vi "Mcp2210 Set Permanent Lock.vi"(8 "error in (no error)":errorcluster, 11 "handle":i32) -> (0 "error out":errorcluster, 3 "handle out":i32)   [LabVIEW 2015, in "mcp2210.lvlib"]
doc: "Permanently locks the device NVRAM settings.\n!!!!!!!!!!!!!!!!!!!!!!!!!!!!!!!! WARNING !!!!!!!!!!!!!!!!!!!!!!!!!!!!!!!!!!!\nUSE THIS FUNCTION WITH GREAT CAUTION. THERE IS NO WAY TO REMOVE THE PERMANENT LOCK\nTHE CHIP POWER-UP DEFAULT SETTINGS CANNOT BE CHANGED AFTER THIS FUNCTION CALL\n!!!!!!!!!!!!!!!!!!!!!!!!!!!!!!!!!!!!!!!!!!!!!!!!!!!!!!!!!!!!!!!!!!!!!!!!!!!!!!!!!!\nThe function returns 0 (M_E_SUCCESS) if the lock configuration is accepted\nor negative error code in case of device communication failure or if the access control configuration\nchange is not accepted by the device.\nError codes in case of rejected configuration change:\n- M_E_ERR_NVRAM_LOCKED - NVRAM is already permanently locked\n- M_E_ERR_BLOCKED_ACCESS - NVRAM is password protected. NVRAM change protection must be\ndeactivated first, using M_Mcp2210_EnterPassword() or\nM_Mcp2210_SetAccessControl()\nParameters:\nInputs:\n- IntPtr handle - The USB device handle. Cannot be NULL.\nOutputs:\n- none\nReturns:\n- 0 for success: M_E_SUCCESS\n- negative error code: M_E_ERR_NULL, M_E_ERR_INVALID_HANDLE_VALUE, M_E_ERR_INVALID_PARAMETER\nM_E_ERR_HID_TIMEOUT, M_E_ERR_HID_RW_FILEIO, M_E_ERR_UNKOWN_ERROR\nM_E_ERR_NVRAM_LOCKED, M_E_ERR_BLOCKED_ACCESS\nM_E_ERR_CMD_ECHO, M_E_ERR_CMD_FAILED\n\nMCP2210_DLL_UM_API int __stdcall Mcp2210_SetPermanentLock(void *handle);"
uses:
  <userlib>/mcp2210/mcp2210.lvlib
  <userlib>/mcp2210/mcp2210_dll_um_x86.dll
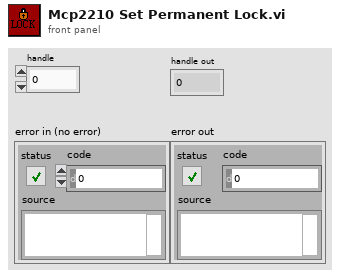
[diagram p1: front panel]
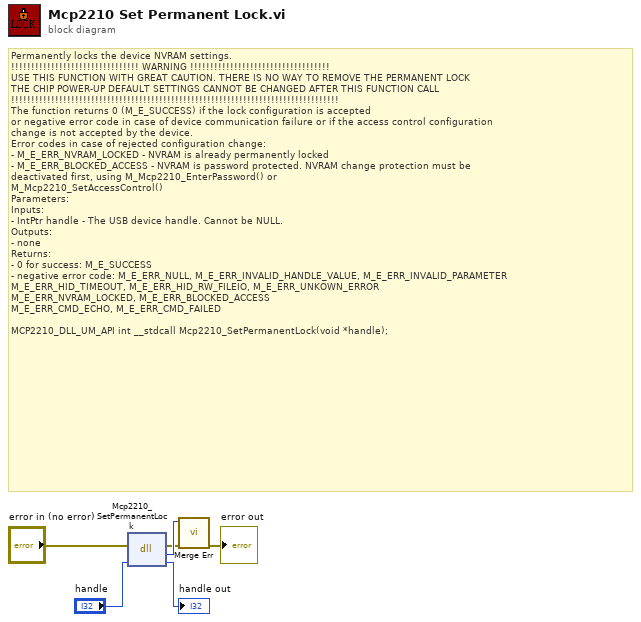
[diagram p0: block diagram]
diagram:
  # "Permanently locks the device NVRAM settings.\n!!!!!!!!!!!!!!!!!!!!!!!!!!!!!!!! WARNING !!!!!!!!!!!!!!!!!!!!!!!!!!!!!!!!!!!\nUSE THIS FUNCTION WITH GREAT CAUTION. THERE IS NO WAY TO REMOVE THE PERMANENT LOCK\nTHE CHIP POWER-UP DEFAULT SETTINGS CANNOT BE CHANGED AFTER THIS FUNCTION CALL\n!!!!!!!!!!!!!!!!!!!!!!!!!!!!!!!!!!!!!!!!!!!!!!!!!!!!!!!!!!!!!!!!!!!!!!!!!!!!!!!!!!\nThe function returns 0 (M_E_SUCCESS) if the lock configuration is accepted\nor negative error code in case of device communication failure or if the access control configuration\nchange is not accepted by the device.\nError codes in case of rejected configuration change:\n- M_E_ERR_NVRAM_LOCKED - NVRAM is already permanently locked\n- M_E_ERR_BLOCKED_ACCESS - NVRAM is password protected. NVRAM change protection must be\ndeactivated first, using M_Mcp2210_EnterPassword() or\nM_Mcp2210_SetAccessControl()\nParameters:\nInputs:\n- IntPtr handle - The USB device handle. Cannot be NULL.\nOutputs:\n- none\nReturns:\n- 0 for success: M_E_SUCCESS\n- negative error code: M_E_ERR_NULL, M_E_ERR_INVALID_HANDLE_VALUE, M_E_ERR_INVALID_PARAMETER\nM_E_ERR_HID_TIMEOUT, M_E_ERR_HID_RW_FILEIO, M_E_ERR_UNKOWN_ERROR\nM_E_ERR_NVRAM_LOCKED, M_E_ERR_BLOCKED_ACCESS\nM_E_ERR_CMD_ECHO, M_E_ERR_CMD_FAILED\n\nMCP2210_DLL_UM_API int __stdcall Mcp2210_SetPermanentLock(void *handle);"
  n1 = dll-call lib="D:/LabVIEW 2015/user.lib/mcp2210/mcp2210_dll_um_x86.*" fn="Mcp2210_SetPermanentLock"(error in="error in (no error)", "handle"="handle") -> (error out=w3:errorcluster, "return type"=w4:i32, "handle"=→"handle out":i32)  [unwired: 2 in, 1 out]
  n2 = call <userlib>:"Merge Err.vi"("error in (no error)"=w3, "return type"=w4) -> ("error out"=→"error out":errorcluster)  [unwired: 9 in]
